vi "Fetch Trace (Occupied Bandwidth).vi"(0 "VISA resource name":refnum<visa-resource-name>, 5 "Timeout (10000 ms)":i32=10000 format="%.0g", 11 "error in (no error)":errorcluster) -> (4 "VISA resource name out":refnum<visa-resource-name>, 6 "Initial X":dbl, 8 "X Increment":dbl, 10 "Trace Array":dbl[](array[numeric]), 15 "error out":errorcluster)   [LabVIEW 2014, in "Agilent MXA Series.lvlib"]
doc: "Fetches trace from the spectrum analyzer (Occupied Bandwidth) and does not initiate data acquisition.\n\n<B>Note:</B>\n\nUse this VI only with other low-level VIs. The high-level VIs automatically incorporate this functionality. This VI does not check the instrument status."
uses:
  Agilent MXA Series.lvlib
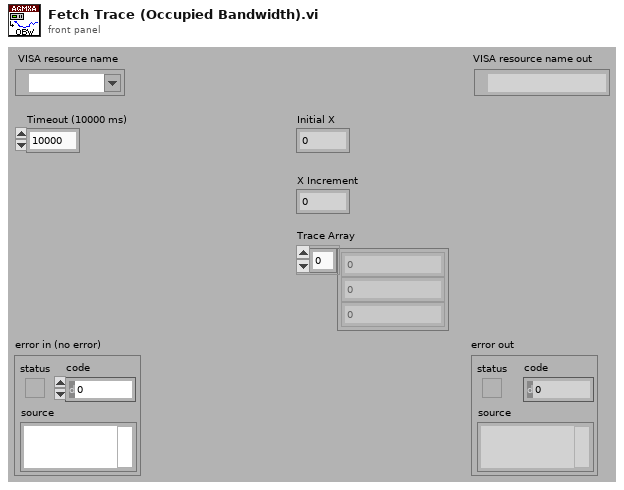
[diagram p1: front panel]
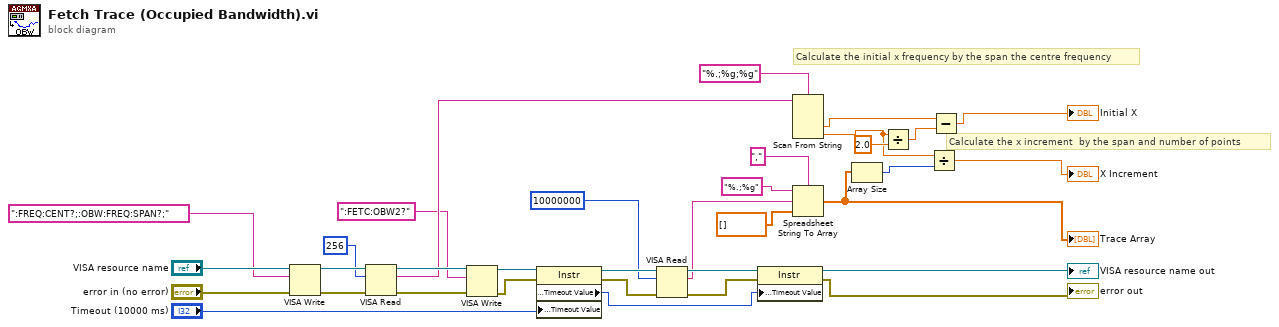
[diagram p0: block diagram]
diagram:
  # "Calculate the x increment  by the span and number of points"
  # "Calculate the initial x frequency by the span the centre frequency"
  n1 = VISA Write(VISA resource name="VISA resource name", write buffer=":FREQ:CENT?;:OBW:FREQ:SPAN?;", error in (no error)="error in (no error)") -> (VISA resource name out=w34:refnum<visa-resource-name>, error out=w33:errorcluster)  [unwired: 1 out]
  n2 = VISA Read(VISA resource name=w34, byte count=256, error in (no error)=w33) -> (VISA resource name out=w21:refnum<visa-resource-name>, read buffer=w19:string, error out=w20:errorcluster)  [unwired: 1 out]
  n3 = VISA Write(VISA resource name=w21, write buffer=":FETC:OBW2?", error in (no error)=w20) -> (VISA resource name out=w26:refnum<visa-resource-name>, error out=w25:errorcluster)  [unwired: 1 out]
  n4 = property on="Property Node" class="Instr"(reference=w26, error in=w25, "General Settings:Timeout Value"="Timeout (10000 ms)") -> (reference out=w31:refnum<visa-resource-name>, error out=w30:errorcluster, "General Settings:Timeout Value"=w27:u32)
  n5 = VISA Read(VISA resource name=w31, byte count=10000000, error in (no error)=w30) -> (VISA resource name out=w29:refnum<visa-resource-name>, read buffer=w5:string, error out=w28:errorcluster)  [unwired: 1 out]
  n6 = property on="Property Node" class="Instr"(reference=w29, error in=w28, "General Settings:Timeout Value"=w27) -> (reference out=→"VISA resource name out":refnum<visa-resource-name>, error out=→"error out":errorcluster)
  n7 = Scan From String(format string="%.;%g;%g", input string=w19) -> (output 1=w23:dbl, output 2=w1:dbl)  [unwired: 4 in, 3 out]
  n8 = Spreadsheet String To Array(delimiter (Tab)=",", format string="%.;%g", spreadsheet string=w5, array type (2D Dbl)=dbl[] []) -> (array=w2:dbl[])
  "Trace Array" <- w2
  n9 = Array Size(array=w2) -> (size(s)=w6:i32)
  n10 = Divide(x=w1, y=2.0) -> (x/y=w22:dbl)
  n11 = Divide(x=w1, y=w6) -> (x/y=→"X Increment":dbl)
  n12 = Subtract(x=w23, y=w22) -> (x-y=→"Initial X":dbl)
